vi "Send_Email_Attach_LV82.vi"() -> ()   [LabVIEW 2015, in "StmpEmail.lvclass"]
uses:
  StmpEmail.lvclass
panel:
  in  "Attachment Path":path=path "E:/LabVIEW相关/研究所培训计划/FirstDay/Demo1/src/Demo4/1. 视觉采集工具包的使用.vi"
  in  "From: (email@site.com)":string="qianlingf@gmail.com"
  in  "Port":i32=25
  in  "SMTP Outgoing Mail Server":string="smtp.gmail.com"
  in  "Body:":string="asda"
  in  "Subject:":string="asd"
  in  "To: (email@site.com)":string="923371272@qq.com"
  in  "Email Account Password":string="1110810220"
  in  "Email Account ID":string="qianlingf@gmail.com"
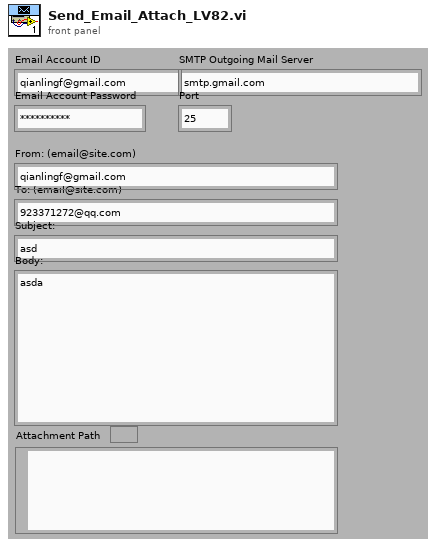
[diagram p1: front panel]
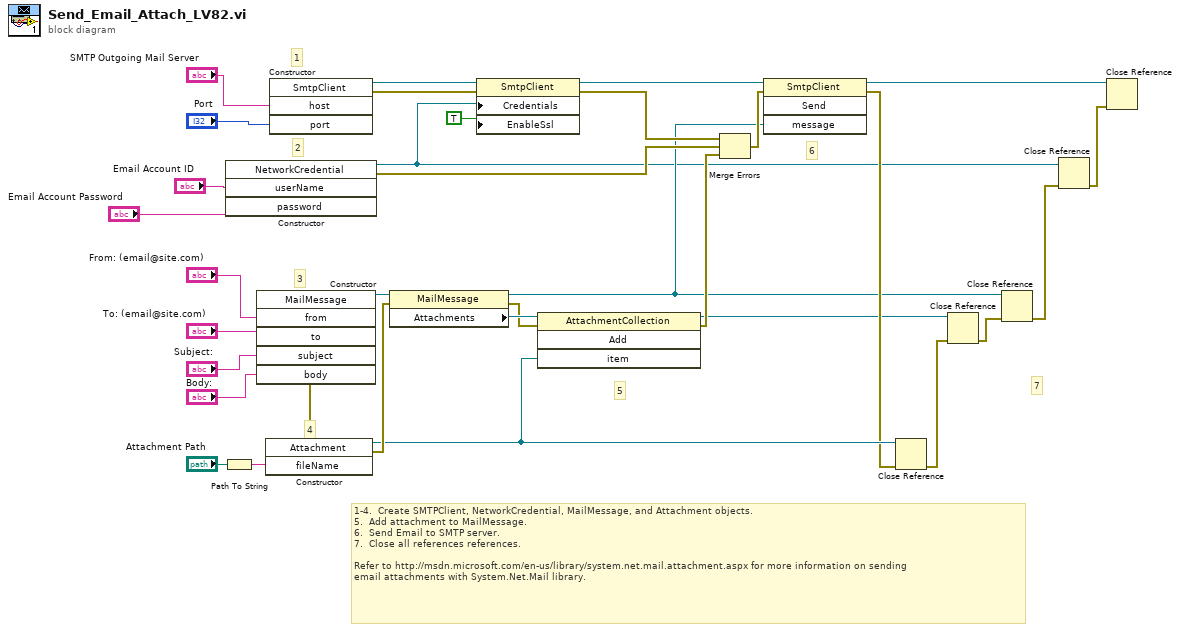
[diagram p0: block diagram]
diagram:
  # "1-4.  Create SMTPClient, NetworkCredential, MailMessage, and Attachment objects.\n5.  Add attachment to MailMessage.\n6.  Send Email to SMTP server.\n7.  Close all references references.\n\nRefer to http://msdn.microsoft.com/en-us/library/system.net.mail.attachment.aspx for more information on sending\nemail attachments with System.Net.Mail library."
  # "7"
  # "6"
  # "5"
  # "4"
  # "3"
  # "2"
  # "1"
  n1 = Path To String(path="Attachment Path") -> (string=w21:string)
  n2 = constructor class="NetworkCredential"("userName"="Email Account ID", "password"="Email Account Password") -> (reference out=w2:refnum<k24>, error out=w12:errorcluster)  [unwired: 3 in, 3 out]
  n3 = constructor class="MailMessage"("from"="From: (email@site.com)", "to"="To: (email@site.com)", "subject"="Subject:", "body"="Body:") -> (reference out=w20:refnum<k24>, error out=w11:errorcluster)  [unwired: 3 in, 5 out]
  n4 = constructor class="Attachment"(error in=w11, "fileName"=w21) -> (reference out=w9:refnum<k24>, error out=w18:errorcluster)  [unwired: 2 in, 2 out]
  n5 = constructor class="SmtpClient"("host"="SMTP Outgoing Mail Server", "port"="Port") -> (reference out=w33:refnum<k24>, error out=w16:errorcluster)  [unwired: 3 in, 3 out]
  n6 = property class="MailMessage"(reference=w20, error in=w18) -> (reference out=w4:refnum<k24>, error out=w17:errorcluster, "Attachments"=w19:refnum<k24>)
  n7 = property class="SmtpClient"(reference=w33, error in=w16, "Credentials"=w2, "EnableSsl"=TRUE ("Enable SSL")) -> (reference out=w32:refnum<k24>, error out=w15:errorcluster)
  n8 = invoke class="AttachmentCollection" method="Add"(reference=w19, error in=w17, "item"=w9) -> (reference out=w7:refnum<k24>, error out=w10:errorcluster)  [unwired: 1 in, 2 out]
  n9 = Merge Errors(w15, w12, w10) -> (w14:errorcluster)
  n10 = invoke class="SmtpClient" method="Send"(reference=w32, error in=w14, "message"=w4) -> (reference out=w13:refnum<k24>, error out=w8:errorcluster)  [unwired: 1 in, 2 out]
  n11 = Close Reference(reference=w9, error in (no error)=w8) -> (error out=w6:errorcluster)
  n12 = Close Reference(reference=w7, error in (no error)=w6) -> (error out=w5:errorcluster)
  n13 = Close Reference(reference=w4, error in (no error)=w5) -> (error out=w3:errorcluster)
  n14 = Close Reference(reference=w2, error in (no error)=w3) -> (error out=w1:errorcluster)
  n15 = Close Reference(reference=w13, error in (no error)=w1) -> ()  [unwired: 1 out]
